vi "BotSpeak_Globals.vi"() -> ()   [LabVIEW 2012]
uses:
  <userlib>/BotSpeak/VIs/Direct/BotSpeak_Control.ctl
panel:
  in  "Variable Format":string
  out "Abort?":bool
  in  "Current Buffer":string
  in  "Status String":string
  in  "Last Bot":T1
  out "Silent?":bool
  in  "PacketSize":i32=50
  in  "Comm":T2(array[cluster])
  out "Script Sent":string
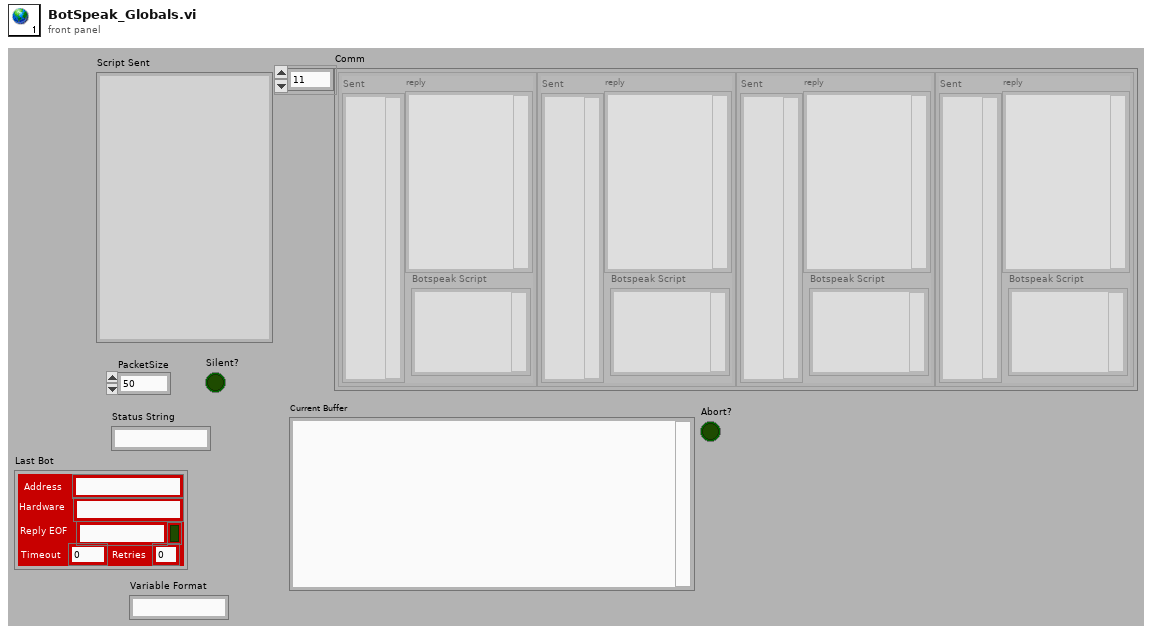
[diagram p1: front panel]
types:
  T1 = typedef "BotSpeak_Control.ctl" = cluster{"Address":string, "Reply EOF":string, "Hardware":string, "Retries":i8, "Timeout":i32, "Open?":bool}
  T2 = cluster{"Sent":string, "reply":string, "Botspeak Script":string}[]
diagram:
